vi "SQL_在指定表中指定字段更新数据.vi"(6 "error in (no error)":errorcluster caption="错误输入（无错误）", 8 "Condition(条件)":string="WHERE 产品型号='%s'", 9 "字段值(字符)":string[](array[string]), 10 "字段名(字符)":string[](array[string]), 11 "表名":string="d7") -> (3 "SQL_在指定表中指定字段更新数据":string, 4 "error out":errorcluster caption="错误输出")   [LabVIEW 2014]
doc: "该模板用于创建子VI。"
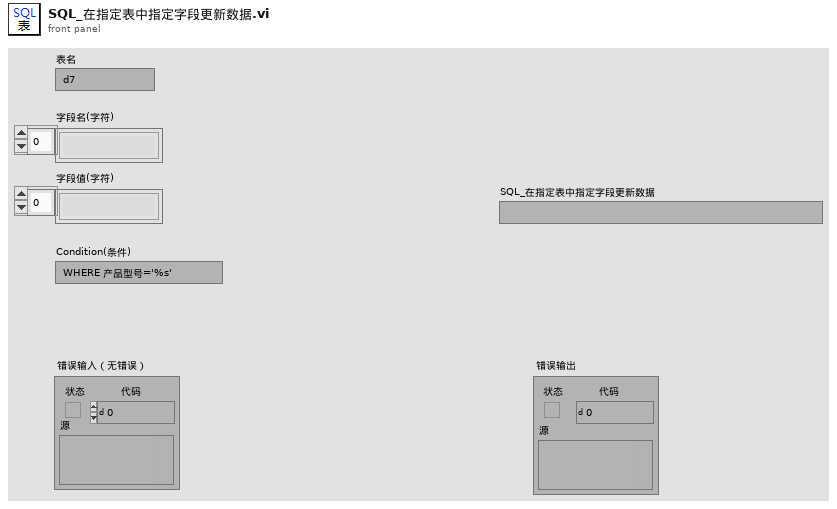
[diagram p1: front panel]
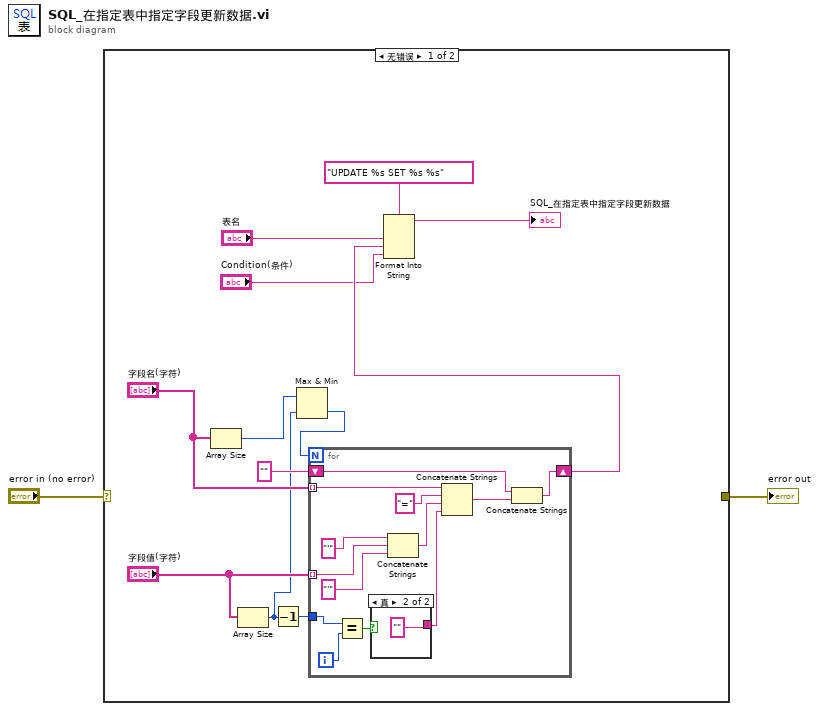
[diagram p0: block diagram]
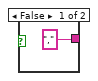
[diagram p2: hidden frame]
diagram:
  n1 = case shown="无错误" "error in (no error)" {
    selector: "error in (no error)" -> [_ w30]
    tunnel: [_ w30] -> w1
    frame No Error {
      n2 = Array Size(array="字段名(字符)") -> (size(s)=w4:i32)
      n3 = Array Size(array="字段值(字符)") -> (size(s)=w3:i32)
      n4 = Decrement(x=w3) -> (x-1=w9:i32)
      n5 = Max & Min(x=w4, y=w3) -> (min(x,y)=w8:i32)  [unwired: 1 out]
      n6 = for {
        N: w8 -> [_]
        tunnel: "字段值(字符)" -> [w27] mode=indexing
        tunnel: w9 -> [w23]
        tunnel: "字段名(字符)" -> [w18] mode=indexing
        shift-right: [w15] -> w6
        shift-left: "" -> [w17]
        i -> [w22]
        n7 = Equal?(x=w23, y=w22) -> (x = y?=w24:bool)
        n8 = case shown="真" w24 {
          tunnel: ["," ""] -> w19
          frame False {
          }
          frame True {
          }
        }
        n9 = Concatenate Strings("'", w27, "'") -> (w20:string)
        n10 = Concatenate Strings(w18, "=", w20, w19) -> (w16:string)
        n11 = Concatenate Strings(w17, w16) -> (w15:string)
      }
      n12 = Format Into String(format string="UPDATE %s SET %s %s", "表名", w6, "Condition(条件)") -> (resulting string=→"SQL_在指定表中指定字段更新数据":string)  [unwired: 2 in, 1 out]
    }
    frame Error {
    }
  }
  "error out" <- w1
